vi "Process Raw CAN TDMS into Usable TDMS.vi"(9 "Destination":path, 11 "Source":path) -> ()   [LabVIEW 2014]
uses:
  <vilib>/RioEmbeddedCAN/RioEmbeddedCAN.llb/CANFrameControl.ctl
  8byte to 4 2byte.vi
  TDMS Timestamp and Data.vi
  TDMS Timestamp and Data Double.vi
  BMS/Scale Cell Voltage.vi
  BMS/Scale Cell Temp.vi
panel:
  out "error out 2":errorcluster
  out "error out":errorcluster
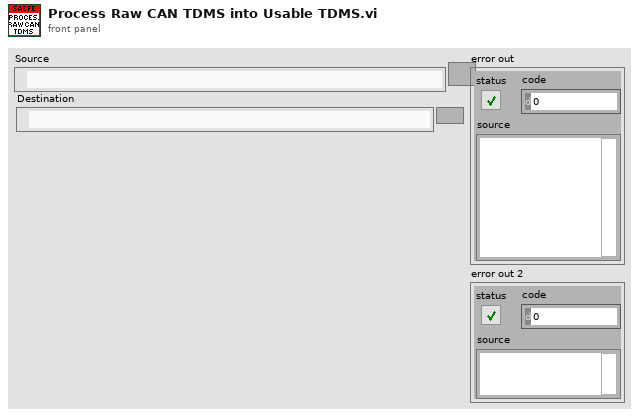
[diagram p1: front panel]
types:
  T1 = enum16{"open", "open or create", "create or replace", "create", "open (read-only)"}
  T2 = typedef "CANFrameControl.ctl" = cluster{"identifier":u32, "extended?":bool, "type":u8, "payload":u8[]}
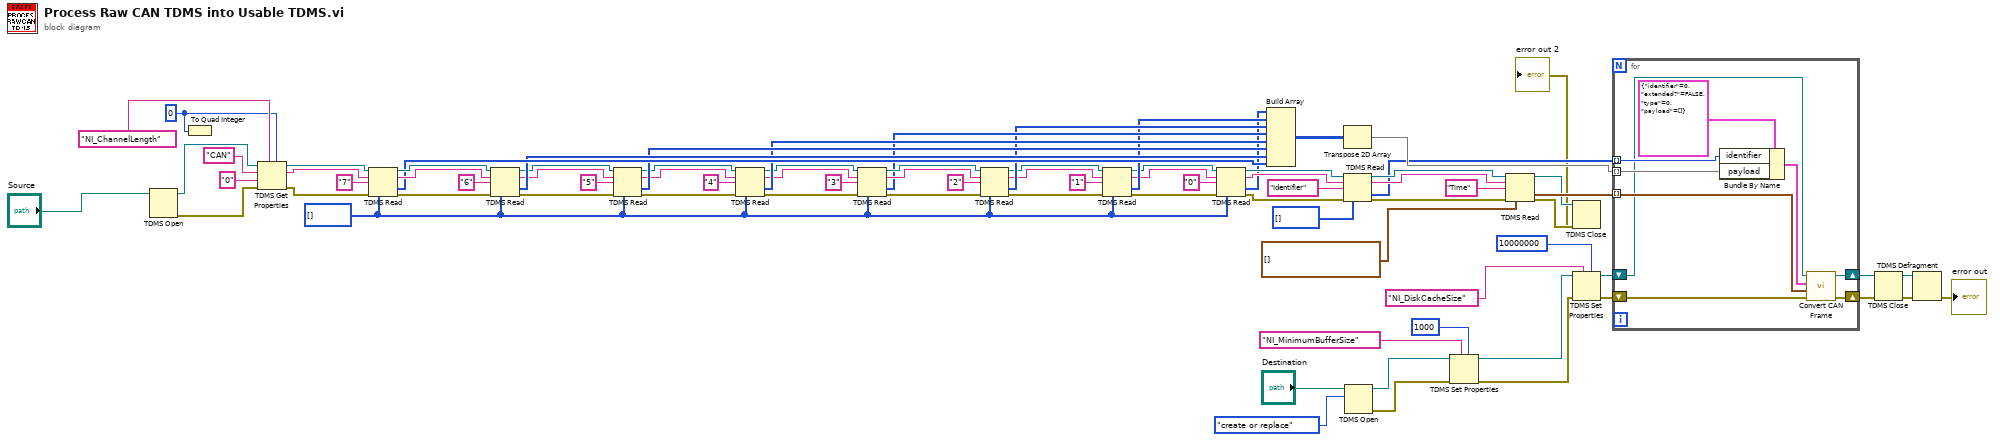
[diagram p0: block diagram]
diagram:
  w9 = u8[] []
  w76 = u64 0 ("data type")
  n1 = TDMS Open(11:"Source") -> (0:w81:errorcluster, 3:w82:refnum<k34>)  [unwired: 6 in]
  n2 = To Quad Integer(1:w76) -> ()  [unwired: 1 out]
  n3 = TDMS Get Properties(5:w76, 7:"NI_ChannelLength" ("property name"), 8:w81, 9:"0" ("channel name"), 10:"CAN" ("group name"), 11:w82) -> (0:w74:errorcluster, 2:w73:string, 3:w75:refnum<k34>)  [unwired: 3 out]
  n4 = TDMS Read(0:w75, 5:w73, 7:"7" ("channel name(s) in"), 11:w74, 12:w9) -> (4:w71:refnum<k34>, 6:w69:string, 10:w67:u8[], 15:w70:errorcluster)  [unwired: 3 in, 2 out]
  n5 = TDMS Read(0:w71, 5:w69, 7:"6" ("channel name(s) in"), 11:w70, 12:w9) -> (4:w65:refnum<k34>, 6:w63:string, 10:w66:u8[], 15:w64:errorcluster)  [unwired: 3 in, 2 out]
  n6 = TDMS Read(0:w65, 5:w63, 7:"5" ("channel name(s) in"), 11:w64, 12:w9) -> (4:w60:refnum<k34>, 6:w59:string, 10:w61:u8[], 15:w57:errorcluster)  [unwired: 3 in, 2 out]
  n7 = TDMS Read(0:w60, 5:w59, 7:"4" ("channel name(s) in"), 11:w57, 12:w9) -> (4:w55:refnum<k34>, 6:w53:string, 10:w56:u8[], 15:w54:errorcluster)  [unwired: 3 in, 2 out]
  n8 = TDMS Read(0:w55, 5:w53, 7:"3" ("channel name(s) in"), 11:w54, 12:w9) -> (4:w51:refnum<k34>, 6:w49:string, 10:w46:u8[], 15:w50:errorcluster)  [unwired: 3 in, 2 out]
  n9 = TDMS Read(0:w51, 5:w49, 7:"2" ("channel name(s) in"), 11:w50, 12:w9) -> (4:w11:refnum<k34>, 6:w5:string, 10:w45:u8[], 15:w10:errorcluster)  [unwired: 3 in, 2 out]
  n10 = TDMS Read(0:w11, 5:w5, 7:"1" ("channel name(s) in"), 11:w10, 12:w9) -> (4:w4:refnum<k34>, 6:w2:string, 10:w8:u8[], 15:w3:errorcluster)  [unwired: 3 in, 2 out]
  n11 = TDMS Read(0:w4, 5:w2, 7:"0" ("channel name(s) in"), 11:w3, 12:w9) -> (4:w44:refnum<k34>, 6:w42:string, 10:w7:u8[], 15:w43:errorcluster)  [unwired: 3 in, 2 out]
  n12 = Build Array(w7, w8, w45, w46, w56, w61, w66, w67) -> (w34:u8[][])
  n13 = Transpose 2D Array(2D array=w34) -> (transposed array=w33:u8[][])
  n14 = TDMS Read(0:w44, 5:w42, 7:"Identifier" ("channel name(s) in"), 11:w43, 12:u32[] []) -> (4:w39:refnum<k34>, 6:w37:string, 10:w31:u32[], 15:w38:errorcluster)  [unwired: 3 in, 2 out]
  n15 = TDMS Open(10:T1."create or replace" ("operation (0:open)"), 11:"Destination") -> (0:w27:errorcluster, 3:w28:refnum<k34>)  [unwired: 5 in]
  n16 = TDMS Set Properties(5:u32 1000, 7:"NI_MinimumBufferSize", 8:w27, 11:w28) -> (0:w23:errorcluster, 3:w24:refnum<k34>)  [unwired: 2 in, 2 out]
  n17 = TDMS Read(0:w39, 5:w37, 7:"Time" ("channel name(s) in"), 11:w38, 12:timestamp[] []) -> (4:w13:refnum<k34>, 10:w32:timestamp[], 15:w12:errorcluster)  [unwired: 3 in, 3 out]
  n18 = TDMS Close(8:w12, 11:w13) -> (0:→"error out 2":errorcluster)  [unwired: 1 out]
  n19 = TDMS Set Properties(5:u32 10000000, 7:"NI_DiskCacheSize", 8:w23, 11:w24) -> (0:w19:errorcluster, 3:w20:refnum<k34>)  [unwired: 2 in, 2 out]
  n20 = for {
    tunnel: w33 -> [w88] mode=indexing
    tunnel: w32 -> [w89] mode=indexing
    tunnel: w31 -> [w87] mode=indexing
    shift-right: [w83] -> w17
    shift-left: w20 -> [w86]
    shift-right: [w84] -> w18
    shift-left: w19 -> [w85]
    n21 = Bundle By Name(cluster=T2 {"identifier"=0, "extended?"=FALSE, "type"=0, "payload"=[]} ("CAN frame"), "identifier"=w87, "payload"=w88) -> (w90:T2)
    n22 = call "Convert CAN Frame.vi"("error in (no error)"=w85, "timestamp"=w89, "CAN frame"=w90, "tdms file"=w86) -> ("error out"=w84:errorcluster, "tdms file out"=w83:refnum<k34>)  [unwired: 6 in]
  }
  n23 = TDMS Close(8:w18, 11:w17) -> (0:w15:errorcluster, 3:w16:path)
  n24 = TDMS Defragment(4:w15, 7:w16) -> (0:→"error out":errorcluster)
